vi "chart axis set num format lv.vi"(8 "error in (no error)":errorcluster, 10 "num_format":string, 11 "axis":u32) -> (0 "error out":errorcluster)   [LabVIEW 8.6]
doc: "void chart_axis_set_num_format_lv(lxw_chart_axis axis, const char *num_format);"
uses:
  pending_lvxlsxwriter/xlsxwriter.dll
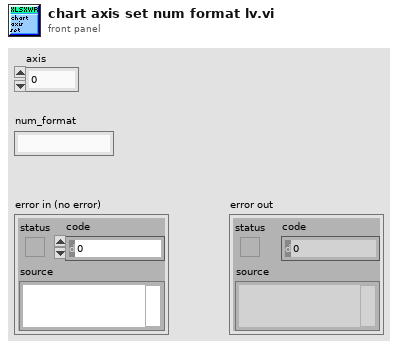
[diagram p1: front panel]
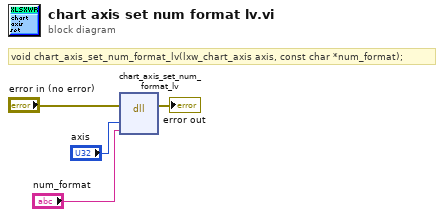
[diagram p0: block diagram]
diagram:
  # "void chart_axis_set_num_format_lv(lxw_chart_axis axis, const char *num_format);"
  n1 = dll-call lib="C:/Users/WDAGUtilityAccount/Desktop/pending_lvxlsxwriter/xlsxwriter.*" fn="chart_axis_set_num_format_lv"(error in="error in (no error)", "axis"="axis", "num_format"="num_format") -> (error out=→"error out":errorcluster)  [unwired: 5 in, 1 out]
